vi "Audio_Transformation_Setted_Frequency_v014.vi"() -> ()   [LabVIEW 2019]
uses:
  <vilib>/sound2/lvsound2.llb/Sound Data Format.ctl
  <vilib>/sound2/lvsound2.llb/Sound Input Read (DBL).vi
  <vilib>/addons/Time Frequency Analysis/Transform.llb/TFA Online Gabor Transform (Real).vi
  <vilib>/addons/_Advanced Signal Processing/NI_AdvSigProcTFA.lvlib
panel:
  out "u(t)":dbl(graph)
  out "V(t)":dbl(graph)
  out "Noise Speech":dbl[](graph)
  in  "Neuron Type":T1(ring)=enum."Phasic Spiking (PS)"
  out "max index(es)":i32
  out "max value":dbl
  out "Waveform Graph":dbl[](graph)
  out "Magnitude of Gabor Coefficients":dbl[][](graph)
  in  "Stop":bool
  # "Step two : Graph of the amplitude of the Gabor coefficient of the different bins"
  # "Step three : Spike Response of the neurons"
  # "Step one: Sound recorded from the computer"
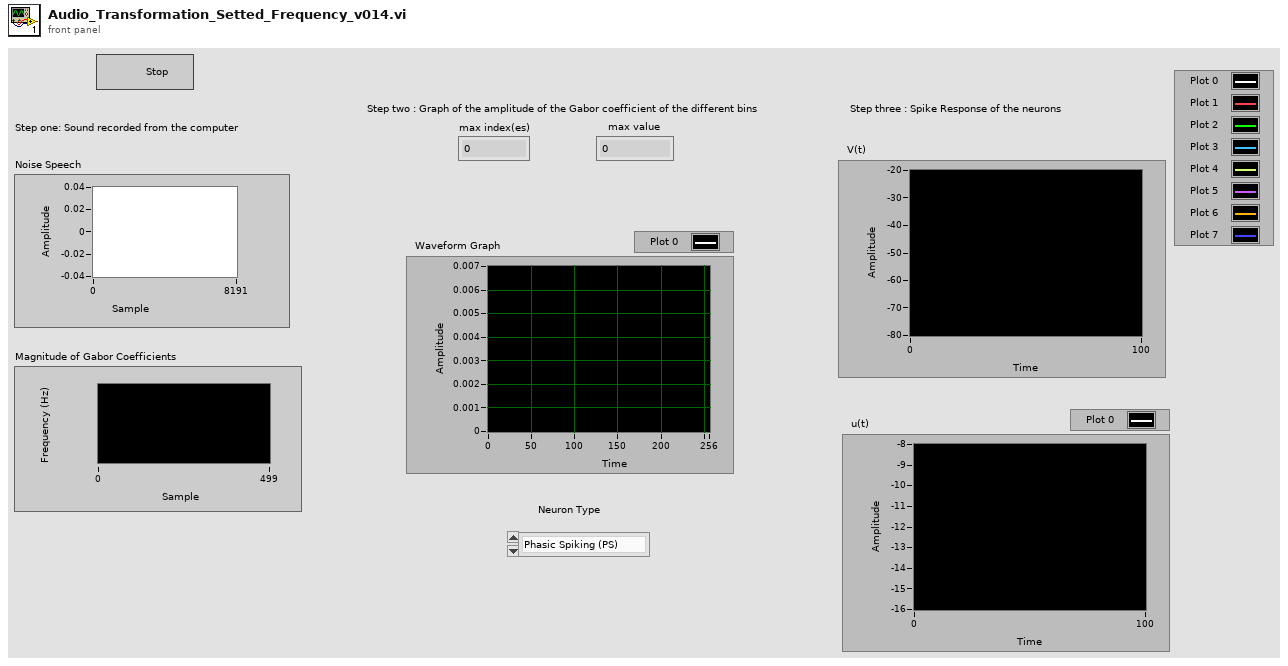
[diagram p1: front panel]
types:
  T1 = enum16{"Regular Spiking (RS)", "Intrinsically Bursting (IB)", "Chattering (CH)", "Fast Spiking (FS)", "Thalamo-Cortical 1 (TC1)", "Thalamo-Cortical 2 (TC2)", "Resonator (RZ)", "Low-Threshold Spiking (LTS)", "Phasic Spiking (PS)"}
  T2 = typedef "Sound Data Format.ctl" = cluster{"sample rate (S/s)":dbl, "number of channels":i32, "bits per sample":i32}
  T3 = cluster{"analysis window":dbl[], "dM (time steps)":i32, "N (frequency bins)":i32}
  T4 = typedef "Sound Input Task ID.ctl" = u32
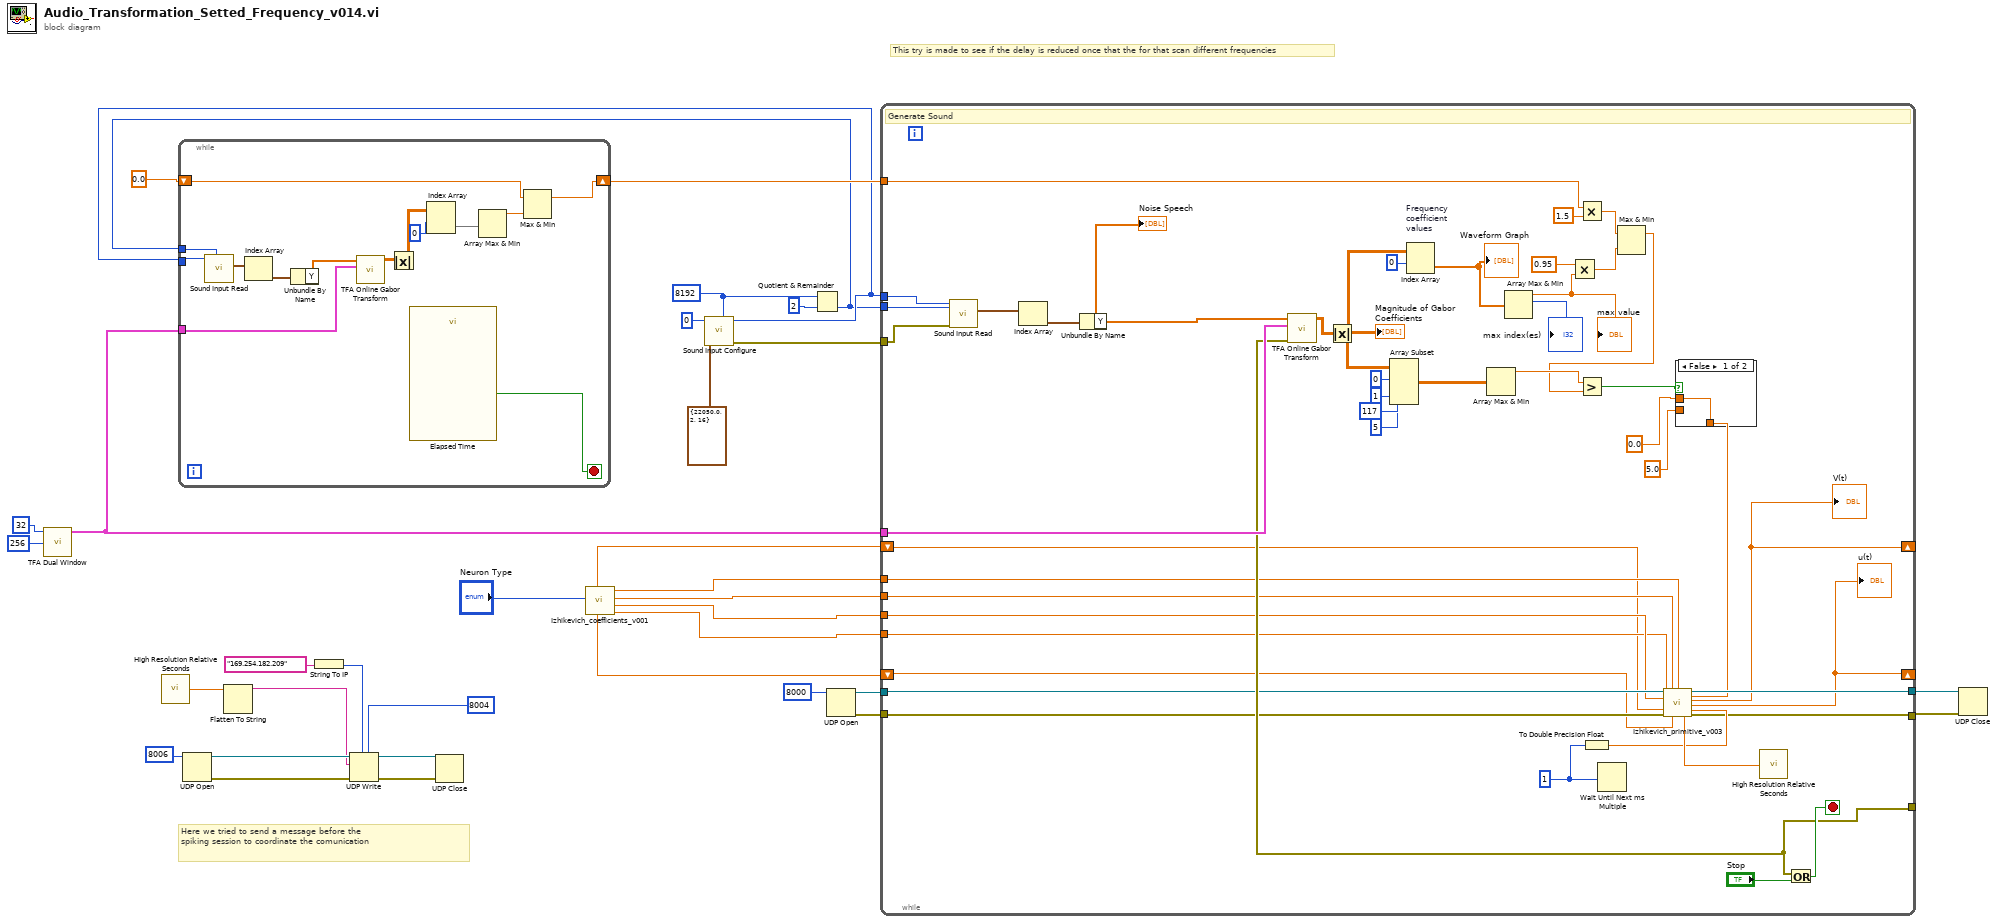
[diagram p0: block diagram]
diagram:
  w23 = 8192 ("number of samples/ch")
  # "This try is made to see if the delay is reduced once that the for that scan different frequencies"
  # "Here we tried to send a message before the\nspiking session to coordinate the comunication"
  n1 = call <vilib>:"TFA Dual Window.vi"("N (frequency bins)"=256, "dM (time steps)"=32) -> ("analysis info"=w20:T3)  [unwired: 7 in, 2 out]
  n2 = call <vilib>:"High Resolution Relative Seconds.vi"() -> ("relative seconds"=w3:dbl)
  n3 = UDP Open(11:u16 8006 ("port")) -> (port=w14:refnum<k16>, 0:w13:errorcluster)  [unwired: 4 in, 1 out]
  n4 = Flatten To String(anything=w3) -> (data string=w9:string)  [unwired: 3 in, 2 out]
  n5 = String To IP(1:"169.254.182.209" ("name")) -> (0:w11:u32)
  n6 = UDP Write(address=w11, port or service name=u16 8004, connection ID=w14, data in=w9, 8:w13) -> (error out=w5:errorcluster, 3:w6:refnum<k16>)  [unwired: 1 in]
  n7 = UDP Close(connection ID=w6, 8:w5) -> ()  [unwired: 2 out]
  n8 = call "Izhikevich_coefficients_v001.vi"("Neuron Type"="Neuron Type") -> ("d"=w28:dbl, "c"=w29:dbl, "b"=w30:dbl, "a"=w31:dbl, "u0"=w1:dbl, "v0"=w2:dbl)  [unwired: 3 in]
  n9 = call <vilib>:"Sound Input Configure.vi"("number of samples/ch"=w23, "sound format"=T2 {"sample rate (S/s)"=22050.0, "number of channels"=2, "bits per sample"=16}, "device ID"=u32 0) -> ("error out"=w21:errorcluster, "task ID"=w17:T4)  [unwired: 7 in]
  n10 = Quotient & Remainder(x=w23, y=2) -> (floor(x/y)=w16:i32)  [unwired: 1 out]
  n11 = while {
    tunnel: w20 -> [w46]
    shift-right: [w38] -> w18
    shift-left: 0.0 -> [w39]
    tunnel: w17 -> [w36]
    tunnel: w16 -> [w35]
    stop <- w37 stop-if-true
    n12 = call-poly <vilib>:"Sound Input Read.vi"("number of samples/ch"=w35, "task ID"=w36) -> ("data"=w47:waveform(dbl)[])  [unwired: 7 in, 2 out]
    n13 = Index Array(array=w47) -> (element=w48:waveform(dbl))  [unwired: 1 in]
    n14 = Unbundle By Name(w48) -> ("Y"=w45:dbl[])
    n15 = call-poly <vilib>:"TFA Online Gabor Transform.vi"("transform info"=w46, "signal"=w45) -> ("Gabor coef"=w44:cdb[][])  [unwired: 7 in, 2 out]
    n16 = Absolute Value(x=w44) -> (abs(x)=w42:dbl[][])
    n17 = call "Elapsed Time"() -> ("Time has Elapsed"=w37:bool)  [unwired: 12 in, 7 out]
    n18 = Index Array(array=w42, index (row)=0) -> (element=w41:dbl[])  [unwired: 1 in]
    n19 = Array Max & Min(array=w41) -> (max value=w40:dbl)  [unwired: 3 out]
    n20 = Max & Min(x=w39, y=w40) -> (max(x,y)=w38:dbl)  [unwired: 1 out]
  }
  n21 = UDP Open(11:u16 8000 ("port")) -> (port=w8:refnum<k16>, 0:w7:errorcluster)  [unwired: 4 in, 1 out]
  n22 = while {
    tunnel: [w88] -> _
    tunnel: w20 -> [w93]
    shift-right: [w49] -> _
    shift-left: w2 -> [w53]
    shift-right: [w50] -> _
    shift-left: w1 -> [w52]
    tunnel: w31 -> [w62]
    tunnel: w30 -> [w63]
    tunnel: w29 -> [w61]
    tunnel: w28 -> [w60]
    tunnel: w8 -> [w64]
    tunnel: w7 -> [w59]
    tunnel: [w56] -> w27
    tunnel: [w57] -> w26
    tunnel: w17 -> [w85]
    tunnel: w21 -> [w84]
    tunnel: w16 -> [w86]
    tunnel: w18 -> [w70]
    stop <- w94 stop-if-true
    w87 = u32 1 ("millisecond multiple")
    # "Generate Sound"
    n23 = call-poly <vilib>:"Sound Input Read.vi"("number of samples/ch"=w86, "error in (no error)"=w84, "task ID"=w85) -> ("data"=w82:waveform(dbl)[])  [unwired: 6 in, 2 out]
    n24 = Index Array(array=w82) -> (element=w83:waveform(dbl))  [unwired: 1 in]
    n25 = Unbundle By Name(w83) -> ("Y"=w81:dbl[])
    "Noise Speech" <- w81
    n26 = call-poly <vilib>:"TFA Online Gabor Transform.vi"("transform info"=w93, "signal"=w81) -> ("error out"=w88:errorcluster, "Gabor coef"=w92:cdb[][])  [unwired: 7 in, 1 out]
    n27 = Absolute Value(x=w92) -> (abs(x)=w73:dbl[][])
    "Magnitude of Gabor Coefficients" <- w73
    n28 = Array Subset(array=w73, index (row)=0 ("index"), length (row)=1 ("length"), index (col)=117 ("index"), length (col)=5 ("length")) -> (w76:dbl[][])
    n29 = Index Array "Frequency \ncoefficient \nvalues"(array=w73, index (row)=0) -> (element=w90:dbl[])  [unwired: 1 in]
    "Waveform Graph" <- w90
    n30 = Array Max & Min(array=w76) -> (max value=w75:dbl)  [unwired: 3 out]
    n31 = Array Max & Min(array=w90) -> (max value=w67:dbl, max index (indices)=→"max index(es)":i32)  [unwired: 2 out]
    "max value" <- w67
    n32 = Multiply(x=0.95 ("y"), y=w67) -> (x*y=w68:dbl)
    n33 = Multiply(x=w70, y=1.5) -> (x*y=w69:dbl)
    n34 = To Double Precision Float(number=w87) -> (double precision float=w58:dbl)
    n35 = Wait Until Next ms Multiple(millisecond multiple=w87) -> ()  [unwired: 1 out]
    n36 = Max & Min(x=w69, y=w68) -> (max(x,y)=w72:dbl)  [unwired: 1 out]
    n37 = Greater?(x=w75, y=w72) -> (0:w74:bool)
    n38 = case shown="False" w74 {
      tunnel: 5.0 -> [_ w97]
      tunnel: 0.0 -> [w96 _]
      tunnel: [w96 w97] -> w51
      frame False {
      }
      frame True {
      }
    }
    n39 = call <vilib>:"High Resolution Relative Seconds.vi"() -> ("relative seconds"=w65:dbl)
    n40 = call "Izhikevich_primitive_v003.vi"("UDP Network Connection in"=w64, "b"=w63, "a"=w62, "I"=w51, "c"=w61, "d"=w60, "v(t)"=w53, "Time"=w65, "error in (no error)"=w59, "u(t)"=w52, "dt"=w58) -> ("UDP Network Connection out"=w57:refnum<k16>, "v(t+dt)"=w49:dbl, "u(t+dt)"=w50:dbl, "error out"=w56:errorcluster)  [unwired: 1 in]
    "V(t)" <- w49
    "u(t)" <- w50
    n41 = Or(x=w88, y="Stop") -> (x .or. y?=w94:bool)
  }
  n42 = UDP Close(connection ID=w26, 8:w27) -> ()  [unwired: 2 out]
